vi "CS POLARIS BME DG.ProcEvents.vi"(0 "i ref in":refnum<vi>, 5 "error in (no error)":errorcluster) -> (14 "i ref out":refnum<vi>, 19 "error out":errorcluster)   [LabVIEW 2009, in "CS POLARIS BME DG.lvlib"]
doc: "This method is used to define the events the object will listen to. Add your own events here."
uses:
  CS POLARIS BME DG.lvlib
  CSCore/BaseProcess/BaseProcess.event definition.ctl
  CSCore/CAEObj/CAEObj.event definition.ctl
  CSCore/BaseProcess/BaseProcess.descriptor string definition.ctl
  CSCore/BaseProcess/BaseProcess.lvlib
  CSCore/CAEObj/CAEObj.lvlib
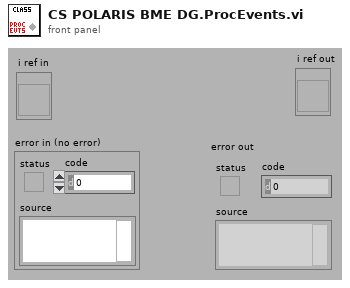
[diagram p1: front panel]
types:
  T1 = typedef "BaseProcess.lvlib/BaseProcess.event definition.ctl" = cluster{"CAEEvtDef":T2, "Data Descriptor":T3}
  T2 = typedef "CAEObj.lvlib/CAEObj.event definition.ctl" = cluster{"URL":string, "enable":bool, "ignoreResID":bool}
  T3 = typedef "BaseProcess.lvlib/BaseProcess.descriptor string definition.ctl" = string
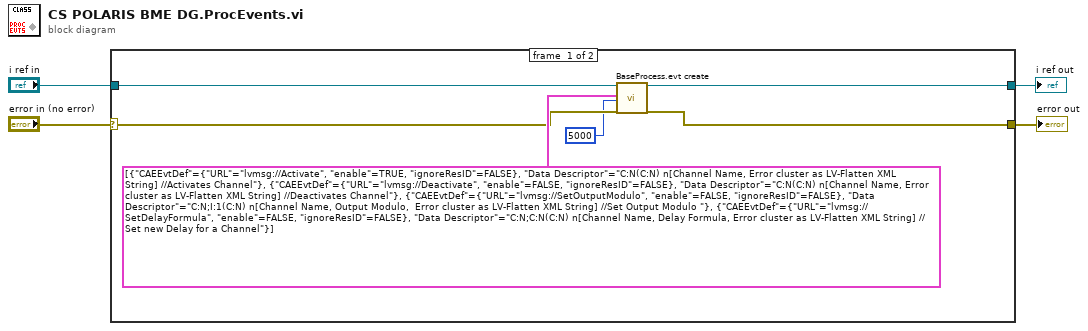
[diagram p0: block diagram]
diagram:
  n1 = case shown="No Error" "error in (no error)" {
    selector: "error in (no error)" -> [w6 w11]
    tunnel: "i ref in" -> [w10 w12]
    tunnel: [w9 w12] -> w3
    tunnel: [w8 w11] -> w2
    frame #0 {
      n2 = call "BaseProcess.evt create.vi"("i ref in"=w10, "newEvents"=T1[] [{"CAEEvtDef"={"URL"="lvmsg://Activate", "enable"=TRUE, "ignoreResID"=FALSE}, "Data Descriptor"="C:N(C:N) n[Channel Name, Error cluster as LV-Flatten XML String] //Activates Channel"}, {"CAEEvtDef"={"URL"="lvmsg://Deactivate", "enable"=FALSE, "ignoreResID"=FALSE}, "Data Descriptor"="C:N(C:N) n[Channel Name, Error cluster as LV-Flatten XML String] //Deactivates Channel"}, {"CAEEvtDef"={"URL"="lvmsg://SetOutputModulo", "enable"=FALSE, "ignoreResID"=FALSE}, "Data Descriptor"="C:N;I:1(C:N) n[Channel Name, Output Modulo,  Error cluster as LV-Flatten XML String] //Set Output Modulo "}, {"CAEEvtDef"={"URL"="lvmsg://SetDelayFormula", "enable"=FALSE, "ignoreResID"=FALSE}, "Data Descriptor"="C:N;C:N(C:N) n[Channel Name, Delay Formula, Error cluster as LV-Flatten XML String] //Set new Delay for a Channel"}] ("new events"), "ms timeout (10000)"=5000, "error in (no error)"=w6) -> ("i ref out"=w9:refnum<vi>, "error out"=w8:errorcluster)  [unwired: 12 in, 2 out]
    }
    frame #1 {
    }
  }
  "i ref out" <- w3
  "error out" <- w2
